vi "High-order Discontinuity Detection.vi"() -> ()   [LabVIEW 2023]
doc: "This example shows how to use the WA Undecimated Wavelet Transform VI to detect high-order discontinuities in an input signal. The input signal is a combination of polynomials (-x^2) and (-x^3). The two polynomials join at index 256. At this point, the signal and its first derivative are continuous but higher-order derivatives are discontinuous. When you use a high-order wavelet to perform the undecimated wavelet transform (UWT), the UWT generates high-amplitude coefficients near the discontinuous point.\n\n<b>Instructions:</b>\n1) Run this VI.\n2) Browse the Block Diagram of this example to learn how to detect high-order discontinuities in a signal by computing the detailed coefficients using the undecimated wavelet transform."
uses:
  <vilib>/addons/Wavelet Analysis/discrete wavelet transform.llb/WA 1D Undecimated Wavelet Transform (Array).vi
  <vilib>/addons/_Advanced Signal Processing/NI_AdvSigProcWA.lvlib
panel:
  out "Detail Coefficients of UWT":dbl[][](graph)
  out "Polynomial (-x^2 concatenated with -x^3)":dbl[](graph)
  # "Overview: Shows how to use the WA Undecimated Wavelet Transform VI to detect high-order discontinuities in an input signal. The input signal is a combination of polynomials (-x^2) and (-x^3). \nRequirements: LabVIEW Full Development System, Advanced Signal Processing Toolkit\nInstructions: \n1. Run this VI.\n2. Browse the Block Diagram of this example to learn how to detect high-order discontinuities in a signal by computing the detailed coefficients using the undecimated wavelet transform."
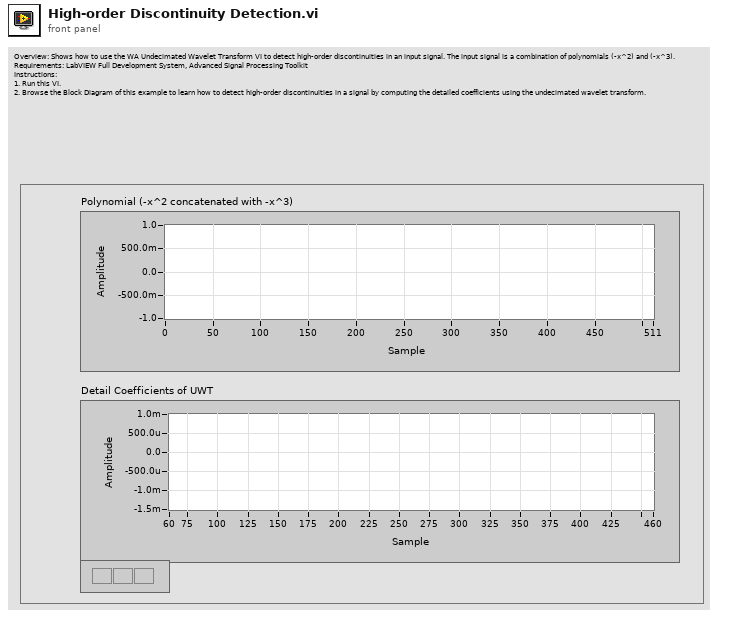
[diagram p1: front panel]
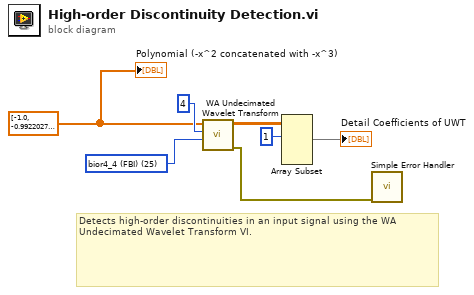
[diagram p0: block diagram]
diagram:
  w2 = dbl[] [-1.0, -0.9922027587890625, -0.98443603515625, -0.9766998291015625, -0.968994140625, -0.9613189697265625, -0.95367431640625, -0.9460601806640625, -0.9384765625, -0.9309234619140625, -0.92340087890625, -0.9159088134765625, -0.908447265625, -0.9010162353515625, -0.89361572265625, -0.8862457275390625, -0.87890625, -0.8715972900390625, -0.86431884765625, -0.8570709228515625, -0.849853515625, -0.8426666259765625, -0.83551025390625, -0.8283843994140625, -0.8212890625, -0.8142242431640625, -0.80718994140625, -0.8001861572265625, -0.793212890625, -0.7862701416015625, -0.77935791015625, -0.7724761962890625, -0.765625, -0.7588043212890625, -0.75201416015625, -0.7452545166015625, -0.738525390625, -0.7318267822265625, -0.72515869140625, -0.7185211181640625, -0.7119140625, -0.7053375244140625, -0.69879150390625, -0.6922760009765625, -0.685791015625, -0.6793365478515625, -0.67291259765625, -0.6665191650390625, -0.66015625, -0.6538238525390625, -0.64752197265625, -0.6412506103515625, -0.635009765625, -0.6287994384765625, -0.62261962890625, -0.6164703369140625, -0.6103515625, -0.6042633056640625, -0.59820556640625, -0.5921783447265625, -0.586181640625, -0.5802154541015625, -0.57427978515625, -0.5683746337890625, -0.5625, -0.5566558837890625, -0.55084228515625, -0.5450592041015625, -0.539306640625, -0.5335845947265625, -0.52789306640625, -0.5222320556640625, -0.5166015625, -0.5110015869140625, -0.50543212890625, -0.4998931884765625, -0.494384765625, -0.4889068603515625, -0.48345947265625, -0.4780426025390625, -0.47265625, -0.4673004150390625, -0.46197509765625, -0.4566802978515625, -0.451416015625, -0.4461822509765625, -0.44097900390625, -0.4358062744140625, -0.4306640625, -0.4255523681640625, -0.42047119140625, -0.4154205322265625, -0.410400390625, -0.4054107666015625, -0.40045166015625, -0.3955230712890625, -0.390625, -0.3857574462890625, -0.38092041015625, -0.3761138916015625, -0.371337890625, -0.3665924072265625, -0.36187744140625, -0.3571929931640625, -0.3525390625, -0.3479156494140625, -0.34332275390625, -0.3387603759765625, -0.334228515625, -0.3297271728515625, -0.32525634765625, -0.3208160400390625, -0.31640625, -0.3120269775390625, -0.30767822265625, -0.3033599853515625, -0.299072265625, -0.2948150634765625, -0.29058837890625, -0.2863922119140625, -0.2822265625, -0.2780914306640625, -0.27398681640625, -0.2699127197265625, -0.265869140625, -0.2618560791015625, -0.25787353515625, -0.2539215087890625, -0.25, -0.2461090087890625, -0.24224853515625, -0.2384185791015625, -0.234619140625, -0.2308502197265625, -0.22711181640625, -0.2234039306640625, -0.2197265625, -0.2160797119140625, -0.21246337890625, -0.2088775634765625, -0.205322265625, -0.2017974853515625, -0.19830322265625, -0.1948394775390625, -0.19140625, -0.1880035400390625, -0.18463134765625, -0.1812896728515625, -0.177978515625, -0.1746978759765625, -0.17144775390625, -0.1682281494140625, -0.1650390625, -0.1618804931640625, -0.15875244140625, -0.1556549072265625, -0.152587890625, -0.1495513916015625, -0.14654541015625, -0.1435699462890625, -0.140625, -0.1377105712890625, -0.13482666015625, -0.1319732666015625, -0.129150390625, -0.1263580322265625, -0.12359619140625, -0.1208648681640625, -0.1181640625, -0.1154937744140625, -0.11285400390625, -0.1102447509765625, -0.107666015625, -0.1051177978515625, -0.10260009765625, -0.1001129150390625, -0.09765625, -0.0952301025390625, -0.09283447265625, -0.0904693603515625, -0.088134765625, -0.0858306884765625, -0.08355712890625, -0.0813140869140625, -0.0791015625, -0.0769195556640625, -0.07476806640625, -0.0726470947265625, -0.070556640625, -0.0684967041015625, -0.06646728515625, -0.0644683837890625, -0.0625, -0.0605621337890625, -0.05865478515625, -0.0567779541015625, -0.054931640625, -0.0531158447265625, -0.05133056640625, -0.0495758056640625, -0.0478515625, -0.0461578369140625, -0.04449462890625, -0.0428619384765625, -0.041259765625, -0.0396881103515625, -0.03814697265625, -0.0366363525390625, -0.03515625, -0.0337066650390625, -0.03228759765625, -0.0308990478515625, -0.029541015625, -0.0282135009765625, -0.02691650390625, -0.0256500244140625, -0.0244140625, -0.0232086181640625, -0.02203369140625, -0.0208892822265625, -0.019775390625, -0.0186920166015625, -0.01763916015625, -0.0166168212890625, -0.015625, -0.0146636962890625, -0.01373291015625, -0.0128326416015625, -0.011962890625, -0.0111236572265625, -0.01031494140625, -0.0095367431640625, -0.0087890625, -0.0080718994140625, -0.00738525390625, -0.0067291259765625, -0.006103515625, -0.0055084228515625, -0.00494384765625, -0.0044097900390625, -0.00390625, -0.0034332275390625, -0.00299072265625, -0.0025787353515625, -0.002197265625, -0.0018463134765625, -0.00152587890625, -0.0012359619140625, -0.0009765625, -0.0007476806640625, -0.00054931640625, -0.0003814697265625, -0.000244140625, -0.0001373291015625, -6.103515625e-05, -1.52587890625e-05, 0.0, -5.960464477539063e-08, -4.76837158203125e-07, -1.6093254089355469e-06, -3.814697265625e-06, -7.450580596923828e-06, -1.2874603271484375e-05, -2.0444393157958984e-05, -3.0517578125e-05, -4.3451786041259766e-05, -5.9604644775390625e-05, -7.933378219604492e-05, -0.000102996826171875, -0.0001309514045715332, -0.00016355514526367188, -0.00020116567611694336, -0.000244140625, -0.00029283761978149414, -0.0003476142883300781, -0.0004088282585144043, -0.000476837158203125, -0.0005519986152648926, -0.0006346702575683594, -0.0007252097129821777, -0.000823974609375, -0.0009313225746154785, -0.0010476112365722656, -0.0011731982231140137, -0.001308441162109375, -0.001453697681427002, -0.0016093254089355469, -0.0017756819725036621, -0.001953125, -0.002142012119293213, -0.002342700958251953, -0.002555549144744873, -0.002780914306640625, -0.0030191540718078613, -0.0032706260681152344, -0.0035356879234313965, -0.003814697265625, -0.004108011722564697, -0.004415988922119141, -0.004738986492156982, -0.005077362060546875, -0.005431473255157471, -0.005801677703857422, -0.006188333034515381, -0.006591796875, -0.007012426853179932, -0.007450580596923828, -0.007906615734100342, -0.008380889892578125, -0.00887376070022583, -0.00938558578491211, -0.009916722774505615, -0.010467529296875, -0.011038362979888916, -0.011629581451416016, -0.012241542339324951, -0.012874603271484375, -0.01352912187576294, -0.014205455780029297, -0.0149039626121521, -0.015625, -0.01636892557144165, -0.017136096954345703, -0.01792687177658081, -0.018741607666015625, -0.0195806622505188, -0.020444393157958984, -0.021333158016204834, -0.022247314453125, -0.023187220096588135, -0.02415323257446289, -0.02514570951461792, -0.026165008544921875, -0.027211487293243408, -0.028285503387451172, -0.02938741445541382, -0.030517578125, -0.03167635202407837, -0.03286409378051758, -0.03408116102218628, -0.035327911376953125, -0.03660470247268677, -0.03791189193725586, -0.03924983739852905, -0.040618896484375, -0.042019426822662354, -0.043451786041259766, -0.04491633176803589, -0.046413421630859375, -0.04794341325759888, -0.04950666427612305, -0.05110353231430054, -0.052734375, -0.05439954996109009, -0.05609941482543945, -0.05783432722091675, -0.059604644775390625, -0.061410725116729736, -0.06325292587280273, -0.06513160467147827, -0.067047119140625, -0.06899982690811157, -0.07099008560180664, -0.07301825284957886, -0.07508468627929688, -0.07718974351882935, -0.07933378219604492, -0.08151715993881226, -0.083740234375, -0.0860033631324768, -0.08830690383911133, -0.09065121412277222, -0.09303665161132812, -0.0954635739326477, -0.09793233871459961, -0.10044330358505249, -0.102996826171875, -0.10559326410293579, -0.10823297500610352, -0.11091631650924683, -0.11364364624023438, -0.11641532182693481, -0.1192317008972168, -0.12209314107894897, -0.125, -0.12795263528823853, -0.1309514045715332, -0.13399666547775269, -0.13708877563476562, -0.14022809267044067, -0.14341497421264648, -0.1466497778892517, -0.149932861328125, -0.153264582157135, -0.1566452980041504, -0.1600753664970398, -0.16355514526367188, -0.16708499193191528, -0.17066526412963867, -0.1742963194847107, -0.177978515625, -0.18171221017837524, -0.18549776077270508, -0.18933552503585815, -0.19322586059570312, -0.19716912508010864, -0.20116567611694336, -0.20521587133407593, -0.209320068359375, -0.21347862482070923, -0.21769189834594727, -0.22196024656295776, -0.22628402709960938, -0.23066359758377075, -0.23509931564331055, -0.2395915389060974, -0.244140625, -0.24874693155288696, -0.25341081619262695, -0.2581326365470886, -0.2629127502441406, -0.2677515149116516, -0.27264928817749023, -0.27760642766952515, -0.282623291015625, -0.28770023584365845, -0.29283761978149414, -0.29803580045700073, -0.3032951354980469, -0.3086159825325012, -0.3139986991882324, -0.31944364309310913, -0.324951171875, -0.3305216431617737, -0.33615541458129883, -0.3418528437614441, -0.3476142883300781, -0.3534401059150696, -0.3593306541442871, -0.36528629064559937, -0.371307373046875, -0.37739425897598267, -0.383547306060791, -0.3897668719291687, -0.3960533142089844, -0.4024069905281067, -0.4088282585144043, -0.41531747579574585, -0.421875, -0.4285011887550354, -0.4351963996887207, -0.44196099042892456, -0.4487953186035156, -0.45569974184036255, -0.462674617767334, -0.4697203040122986, -0.476837158203125, -0.4840255379676819, -0.4912858009338379, -0.49861830472946167, -0.5060234069824219, -0.5135014653205872, -0.5210528373718262, -0.5286778807640076, -0.536376953125, -0.5441504120826721, -0.5519986152648926, -0.55992192029953, -0.5679206848144531, -0.5759952664375305, -0.5841460227966309, -0.5923733115196228, -0.600677490234375, -0.6090589165687561, -0.6175179481506348, -0.6260549426078796, -0.6346702575683594, -0.6433642506599426, -0.652137279510498, -0.6609897017478943, -0.669921875, -0.6789341568946838, -0.6880269050598145, -0.6972004771232605, -0.7064552307128906, -0.7157915234565735, -0.7252097129821777, -0.734710156917572, -0.744293212890625, -0.7539592385292053, -0.7637085914611816, -0.7735416293144226, -0.7834587097167969, -0.7934601902961731, -0.8035464286804199, -0.813717782497406, -0.823974609375, -0.8343172669410706, -0.8447461128234863, -0.855261504650116, -0.8658638000488281, -0.8765533566474915, -0.8873305320739746, -0.8981956839561462, -0.909149169921875, -0.9201913475990295, -0.9313225746154785, -0.9425432085990906, -0.9538536071777344, -0.9652541279792786, -0.9767451286315918, -0.9883269667625427] ("[-x^2 -x^3]")
  w6 = u16 25 items=["db02"=0, "db03"=1, "db04"=2, "db05"=3, "db06"=4, "db07"=5, "db08"=6, "db09"=7, "db10"=8, "db11"=9, "db12"=10, "db13"=11, "db14"=12, "Haar"=13, "bior1_3"=14, "bior1_5"=15, "bior2_2"=16, "bior2_4"=17, "bior2_6"=18, "bior2_8"=19, "bior3_1"=20, "bior3_3"=21, "bior3_5"=22, "bior3_7"=23, "bior3_9"=24, "bior4_4 (FBI)"=25, "bior5_5"=38, "bior6_8"=39, "coif1"=26, "coif2"=27, "coif3"=28, "coif4"=29, "coif5"=30, "sym2"=31, "sym3"=32, "sym4"=33, "sym5"=34, "sym6"=35, "sym7"=36, "sym8"=37] ("wavelet")
  # "Detects high-order discontinuities in an input signal using the WA Undecimated Wavelet Transform VI."
  n1 = call-poly <vilib>:"WA Undecimated Wavelet Transform.vi"("wavelet"=w6, "levels"=4 ("level"), "signal"=w2) -> ("error out"=w1:errorcluster, "UWT coef"=w4:dbl[][])  [unwired: 1 in, 6 out]
  n2 = Array Subset(array=w4, index (row)=1 ("index")) -> (→"Detail Coefficients of UWT":dbl[][])  [unwired: 3 in]
  n3 = call <vilib>:"Simple Error Handler.vi"("error in (no error)"=w1) -> ()  [unwired: 4 in, 5 out]
  "Polynomial (-x^2 concatenated with -x^3)" <- w2
